vi "StandAloneTransient_Keithley2230_PSU_POWER_CYCLE_V1.vi"(8 "error in (no error)":errorcluster, 10 "milliseconds to wait":u32, 11 "VISA Refnum in":refnum<visa-resource-name>) -> (0 "error out":errorcluster)   [LabVIEW 2019]
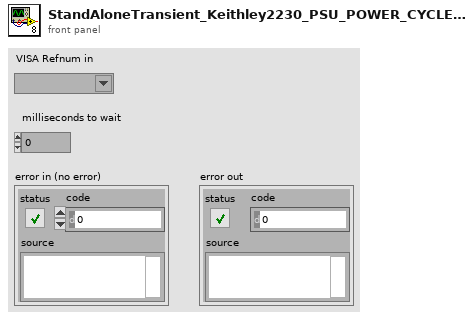
[diagram p1: front panel]
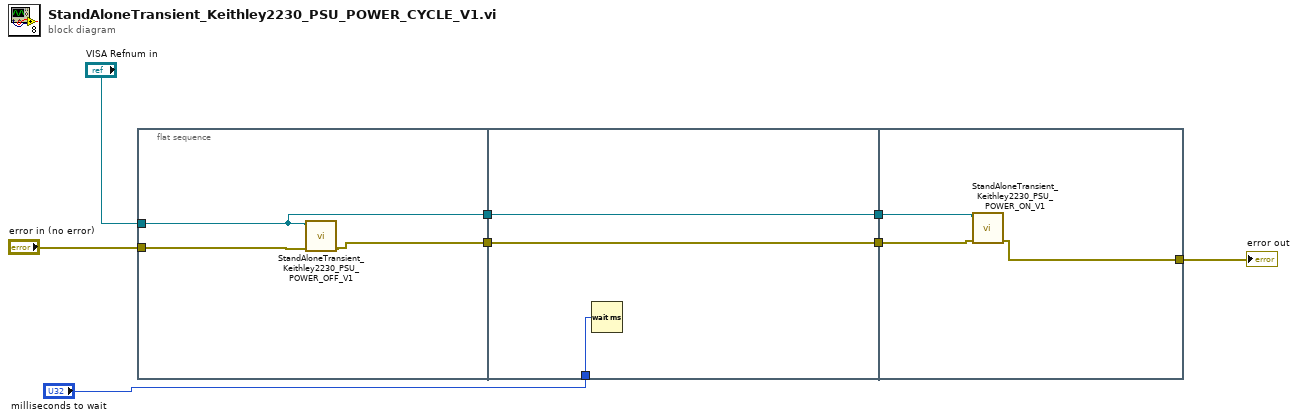
[diagram p0: block diagram]
diagram:
  n1 = flat-sequence {
    tunnel: "VISA Refnum in" -> [w9]
    tunnel: [w9] -> w8
    tunnel: [w11] -> w7
    tunnel: "error in (no error)" -> [w10]
    tunnel: [w14] -> w6
    tunnel: w8 -> [w14]
    tunnel: [w13] -> w5
    tunnel: w7 -> [w13]
    tunnel: "milliseconds to wait" -> [w12]
    tunnel: w6 -> [w15]
    tunnel: w5 -> [w17]
    tunnel: [w16] -> w2
    frame #0 {
      n2 = call "StandAloneTransient_Keithley2230_PSU_POWER_OFF_V1.vi"("error in (no error)"=w10, "VISA resource name"=w9) -> ("error out"=w11:errorcluster)  [unwired: 9 in]
    }
    frame #1 {
      n3 = Wait (ms)(milliseconds to wait=w12) -> ()  [unwired: 1 out]
    }
    frame #2 {
      n4 = call "StandAloneTransient_Keithley2230_PSU_POWER_ON_V1.vi"("error in (no error)"=w17, "VISA resource name"=w15) -> ("error out"=w16:errorcluster)  [unwired: 9 in]
    }
  }
  "error out" <- w2
